vi "CBL Node Check.vi"(5 "TimeOut":u32, 6 "pType":u32, 7 "pVersion":u32, 9 "NodeAddr":u8, 10 "CANIndex":i32, 11 "DevIndex":i32) -> (2 "function return":i32, 3 "pVersion out":u32, 4 "pType out":u32)   [LabVIEW 2010, in "CANBootloader.lvlib"]
doc: "int WINAPI CBL_NodeCheck(int DevIndex,int CANIndex,unsigned char NodeAddr,unsigned int *pVersion,unsigned int *pType,unsigned int TimeOut);"
uses:
  CANBootloader.lvlib
  CANBootloader/Ginkgo_Driver.dll
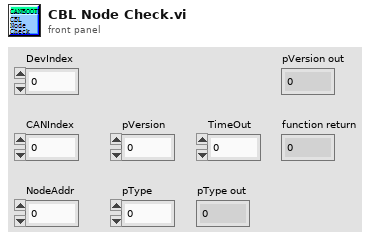
[diagram p1: front panel]
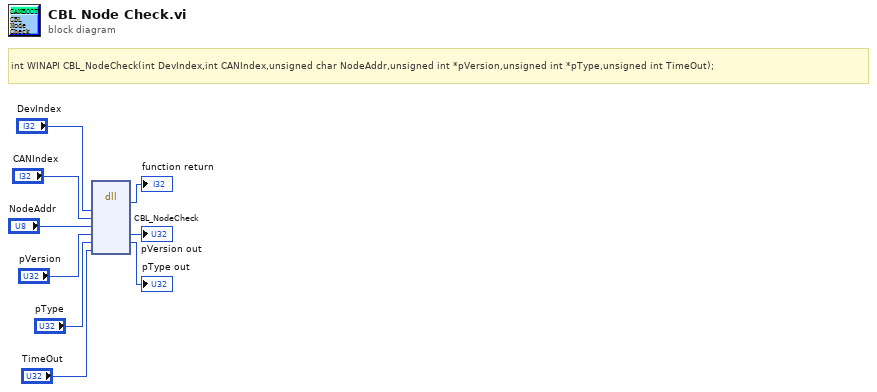
[diagram p0: block diagram]
diagram:
  # "int WINAPI CBL_NodeCheck(int DevIndex,int CANIndex,unsigned char NodeAddr,unsigned int *pVersion,unsigned int *pType,unsigned int TimeOut);"
  n1 = dll-call lib="E:/Project/vt_ginkgo/truck/Ginkgo Driver/vs2010/Ginkgo_USB-I2C&SPI&CAN_API_v2.0.3.3/lib/labview_32bit/CANBootloader/Ginkgo_Driver.*" fn="CBL_NodeCheck"("DevIndex"="DevIndex", "CANIndex"="CANIndex", "NodeAddr"="NodeAddr", "pVersion"="pVersion", "pType"="pType", "TimeOut"="TimeOut") -> (→"function return":i32, "pVersion"=→"pVersion out":u32, "pType"=→"pType out":u32)  [unwired: 7 in, 2 out]
